vi "Resideo Connect.vi"(8 "error in (no error)":errorcluster, 11 "VISA Refnum in":refnum<visa-resource-name>) -> (0 "error out":errorcluster, 3 "Modbus Master out":refnum<class "Modbus Master.lvclass">)   [LabVIEW 2020]
uses:
  <vilib>/NI/Modbus Library/API/Master/Modbus Master.lvclass
  <vilib>/NI/Modbus Library/API/Wrapper/Create Serial Master.vi
  <vilib>/NI/Modbus Library/API/Wrapper/API Main.lvlib
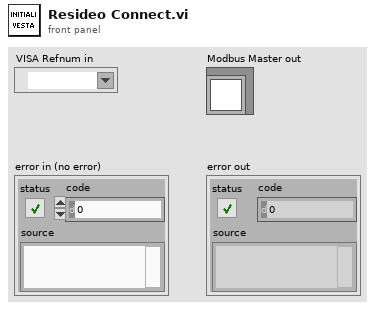
[diagram p1: front panel]
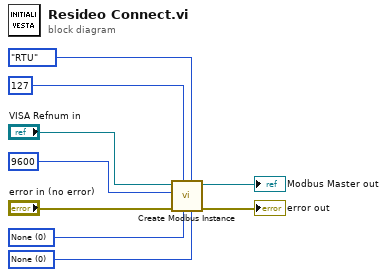
[diagram p0: block diagram]
diagram:
  w7 = u16 0 items=["None", "XON/XOFF", "RTS/CTS", "XON/XOFF & RTS/CTS", "DTR/DSR", "XON/XOFF & DTR/DSR"] ("flow control (none)")
  w6 = u16 0 items=["None", "Odd", "Even", "Mark", "Space"] ("parity (even)")
  n1 = call-poly <vilib>:"Create Modbus Instance.vi"("flow control (none)"=w7, "serial type"=enum16{"RTU", "ASCII"}."RTU", "parity (even)"=w6, "unit ID"=u8 127, "error in"="error in (no error)", "baud rate"=u32 9600, "VISA resource name"="VISA Refnum in") -> ("error out"=→"error out":errorcluster, "serial master instance"=→"Modbus Master out":refnum<class "Modbus Master.lvclass">)  [unwired: 3 in]
